vi "3_Cross_Correlation_Part_II.vi"() -> ()   [LabVIEW 2015]
uses:
  C:/Users/MX-Microscope/Documents/LabVIEW Data/lvoop_campus_2018/Detector_Class/Swabian/time_tagger_vis/TTCSharp32.dll
  TTCSharp32.dll
panel:
  out "Cross correlation showing <60 ps jitter":cluster{"getIndex":i64[], "getData":i32[]}(graph)
  # "cross correlation between channels 0 and 1\nbinwidth=10 ps, n_bins=400, thus we sample 4 ns\nThe standard deviation of the peak\nis the root mean square sum of the\ninput jitters of channels 0 and 1we should see the \ncorrelation delta peaks at a bit more than 1000 ns distance"
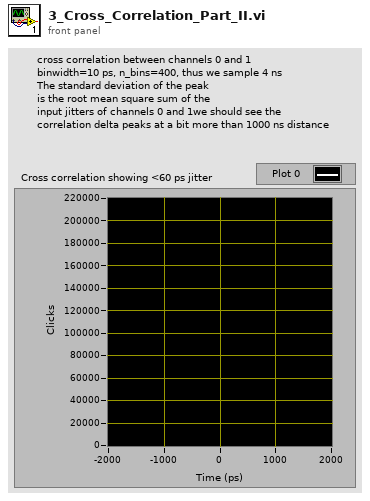
[diagram p1: front panel]
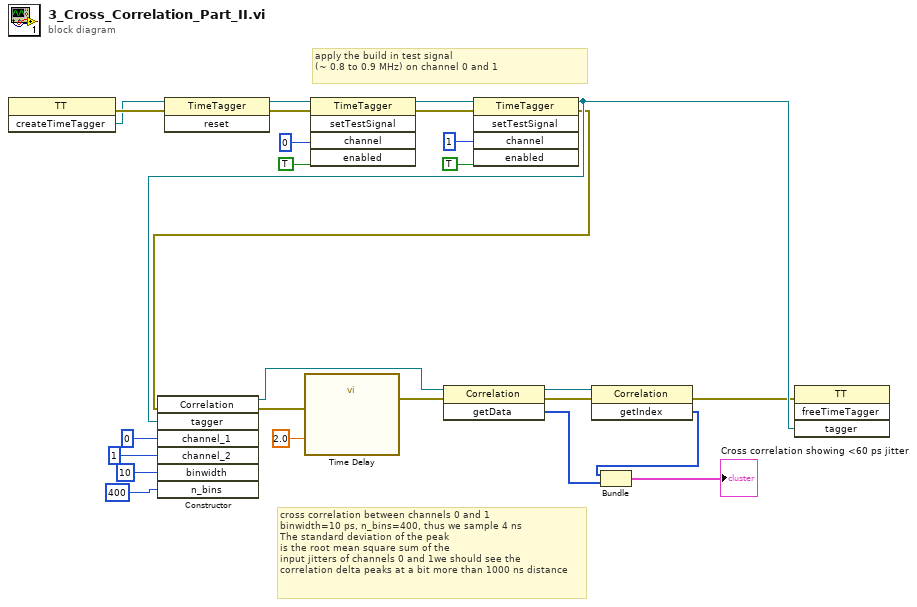
[diagram p0: block diagram]
diagram:
  # "cross correlation between channels 0 and 1\nbinwidth=10 ps, n_bins=400, thus we sample 4 ns\nThe standard deviation of the peak\nis the root mean square sum of the\ninput jitters of channels 0 and 1we should see the \ncorrelation delta peaks at a bit more than 1000 ns distance"
  # "apply the build in test signal\n(~ 0.8 to 0.9 MHz) on channel 0 and 1"
  n1 = invoke class="TT" method="createTimeTagger"() -> (error out=w22:errorcluster, "createTimeTagger"=w21:refnum<k24>)  [unwired: 3 in, 1 out]
  n2 = invoke class="TimeTagger" method="reset"(reference=w21, error in=w22) -> (reference out=w11:refnum<k24>, error out=w12:errorcluster)  [unwired: 1 in, 1 out]
  n3 = invoke class="TimeTagger" method="setTestSignal"(reference=w11, error in=w12, "channel"=u32 0, "enabled"=TRUE) -> (reference out=w13:refnum<k24>, error out=w14:errorcluster)  [unwired: 1 in, 3 out]
  n4 = invoke class="TimeTagger" method="setTestSignal"(reference=w13, error in=w14, "channel"=u32 1, "enabled"=TRUE) -> (reference out=w9:refnum<k24>, error out=w6:errorcluster)  [unwired: 1 in, 3 out]
  n5 = constructor class="Correlation"(error in=w6, "tagger"=w9, "channel_1"=u32 0, "channel_2"=u32 1, "binwidth"=i64 10, "n_bins"=400) -> (reference out=w5:refnum<k24>, error out=w7:errorcluster)  [unwired: 2 in, 6 out]
  n6 = call "Time Delay"("error in (no error)"=w7, "Delay Time (s)"=2.0) -> ("error out"=w8:errorcluster)  [unwired: 9 in]
  n7 = invoke class="Correlation" method="getData"(reference=w5, error in=w8) -> (reference out=w20:refnum<k24>, error out=w19:errorcluster, "getData"=w2:i32[])  [unwired: 1 in]
  n8 = invoke class="Correlation" method="getIndex"(reference=w20, error in=w19) -> (error out=w1:errorcluster, "getIndex"=w3:i64[])  [unwired: 1 in, 1 out]
  n9 = Bundle("getIndex"=w3, "getData"=w2) -> (→"Cross correlation showing <60 ps jitter":cluster{"getIndex":i64[], "getData":i32[]})  [unwired: 1 in]
  n10 = invoke class="TT" method="freeTimeTagger"(error in=w1, "tagger"=w9) -> ()  [unwired: 2 in, 4 out]
